vi "Write.vi"(8 "Error in (no error)":errorcluster, 10 "Log in":T1 {"Priority" items=["EMERGENCY", "ALERT", "CRITICAL", "ERROR", "WARNING", "NOTICE", "INFO", "DEBUG"]}, 11 "LogWriterInterface in":refnum<class "LogWriterInterface.lvclass">) -> (0 "Error out":errorcluster, 3 "LogWriterInterface out":refnum<class "LogWriterInterface.lvclass">)   [LabVIEW 2011, in "LogWriterInterface.lvclass"]
uses:
  LogWriterInterface.lvclass
  Log/LogCluster.ctl
  Log/PrioritiesRing.ctl
  LogWriterInterface.lvclass/LogWriterInterface.ctl
  Filter/LogFilterInterface/LogFilterInterface.lvclass
  Log/Log.lvclass
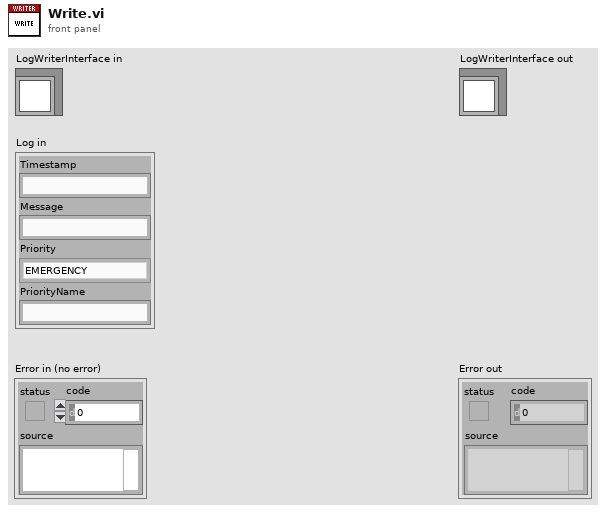
[diagram p1: front panel]
types:
  T1 = typedef "Log.lvclass/LogCluster.ctl" = cluster{"Timestamp":string, "Message":string, "Priority":T2, "PriorityName":string}
  T2 = typedef "Log.lvclass/PrioritiesRing.ctl" = u32
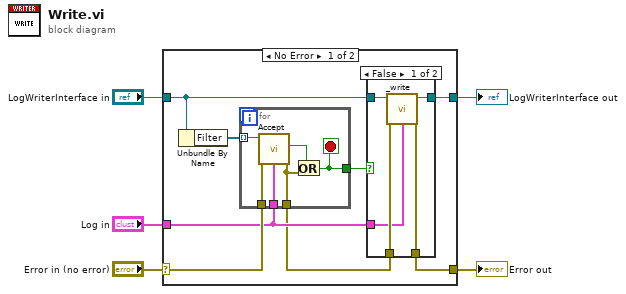
[diagram p0: block diagram]
diagram:
  n1 = case shown="No Error" "Error in (no error)" {
    selector: "Error in (no error)" -> [w12 w27]
    tunnel: [w8 w27] -> w4
    tunnel: [w6 w28] -> w2
    tunnel: "LogWriterInterface in" -> [w7 w28]
    tunnel: "Log in" -> [w10 _]
    frame No Error {
      n2 = Unbundle By Name(w7) -> ("Filter"=w13:refnum<class "LogFilterInterface.lvclass">[])
      n3 = for {
        tunnel: w10 -> [w21]
        tunnel: w13 -> [w26] mode=indexing
        tunnel: w12 -> [w25]
        tunnel: [w23] -> w9
        tunnel: [w22] -> w11
        stop <- w22 stop-if-true
        n4 = call-dynamic "Accept.vi"("Error in (no error)"=w25, "Log in"=w21, "LogFilterInterface in"=w26) -> ("Error out"=w23:errorcluster, "Accept"=w24:bool)  [unwired: 6 in, 1 out]
        n5 = Or(x=w24, y=w23) -> (x .or. y?=w22:bool)
      }
      n6 = case shown="False" w11 {
        tunnel: w10 -> [w14 _]
        tunnel: w9 -> [w16 w19]
        tunnel: [w15 w19] -> w8
        tunnel: w7 -> [w18 w20]
        tunnel: [w17 w20] -> w6
        frame False {
          n7 = call-dynamic "_write.vi"("Error in (no error)"=w16, "Log in"=w14, "LogWriterInterface in"=w18) -> ("Error out"=w15:errorcluster, "LogWriterInterface out"=w17:refnum<class "LogWriterInterface.lvclass">)  [unwired: 7 in]
        }
        frame True {
        }
      }
    }
    frame Error {
    }
  }
  "Error out" <- w4
  "LogWriterInterface out" <- w2
